vi "Replace Stub SubVIs.vi"(8 "error in":errorcluster, 10 "VIs to Process":path[](array[path]), 11 "subVIs to replace":path[](array[path])) -> (0 "error out":errorcluster)   [LabVIEW 2020, in "NIVS_Consolidated_CDW_MetaDataObj.lvclass"]
uses:
  NIVS_Consolidated_CDW_MetaDataObj.lvclass
  <vilib>/Utility/traverseref.llb/TRef TravTarget.ctl
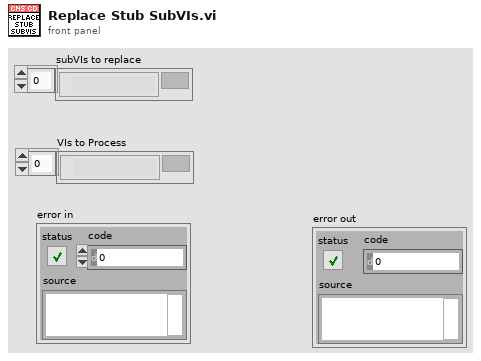
[diagram p1: front panel]
types:
  T1 = typedef "TRef TravTarget.ctl" = enum16{"FP", "BD", "Other"}
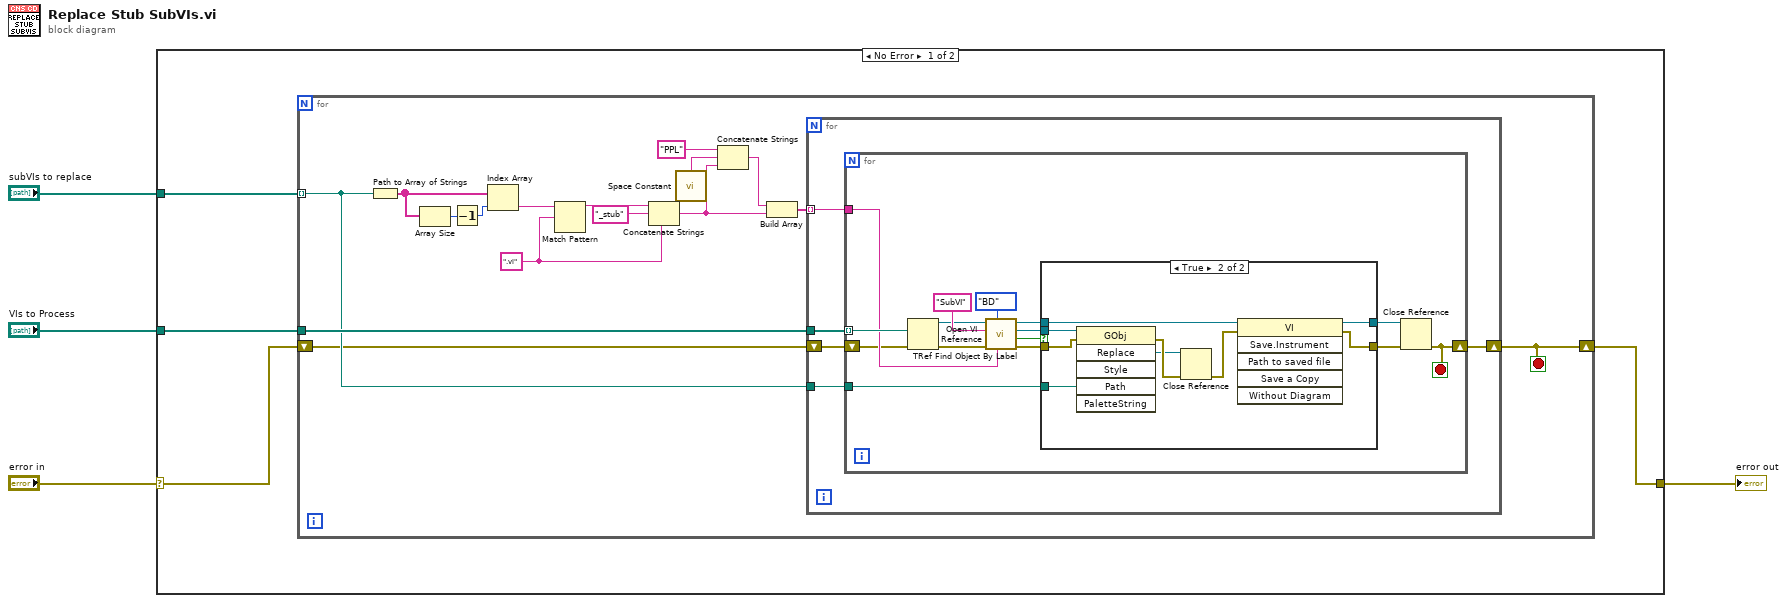
[diagram p0: block diagram]
diagram:
  n1 = case shown="No Error" "error in" {
    selector: "error in" -> [w5 w56]
    tunnel: "VIs to Process" -> [w8 _]
    tunnel: "subVIs to replace" -> [w7 _]
    tunnel: [w6 w56] -> w2
    frame No Error {
      n2 = for {
        tunnel: w7 -> [w16] mode=indexing
        tunnel: w8 -> [w17]
        shift-right: [w14] -> w6
        shift-left: w5 -> [w15]
        stop <- w14 stop-if-true
        w18 = ".vi" ("regular expression")
        n3 = Path to Array of Strings(0:w16) -> (2:w24:string[])  [unwired: 1 out]
        n4 = Array Size(array=w24) -> (size(s)=w23:i32)
        n5 = Decrement(x=w23) -> (x-1=w22:i32)
        n6 = Index Array(array=w24, index=w22) -> (element=w21:string)
        n7 = Match Pattern(string=w21, regular expression=w18) -> (before substring=w20:string)  [unwired: 1 in, 3 out]
        n8 = Concatenate Strings(w20, "_stub" ("string"), w18) -> (w10:string)
        n9 = call <vilib>:"Space Constant.vi"() -> ("String"=w13:string)
        n10 = Concatenate Strings("PPL" ("string"), w13, w10) -> (w11:string)
        n11 = Build Array(w11, w10) -> (w9:string[])
        n12 = for {
          tunnel: w17 -> [w29]
          tunnel: w16 -> [w28]
          shift-right: [w26] -> w14
          shift-left: w15 -> [w27]
          tunnel: w9 -> [w25] mode=indexing
          n13 = for {
            tunnel: w29 -> [w40] mode=indexing
            tunnel: w25 -> [w39]
            tunnel: w28 -> [w36]
            shift-right: [w30] -> w26
            shift-left: w27 -> [w31]
            stop <- w30 stop-if-true
            n14 = Open VI Reference(vi path=w40, error in (no error)=w31) -> (vi reference=w42:refnum<vi>, error out=w41:errorcluster)  [unwired: 4 in]
            n15 = call <vilib>:"TRef Find Object By Label.vi"("Label"=w39, "Traverse Target"=TRef_TravTarget."BD", "error in (no error)"=w41, "Class Name"="SubVI", "VI Ref"=w42) -> ("error out"=w34:errorcluster, "Found?"=w38:bool, "Found Obj Ref"=w37:refnum<vi>, "dup VI Ref"=w35:refnum<vi>)  [unwired: 3 in]
            n16 = case shown="True" w38 {
              tunnel: w37 -> [_ w55]
              tunnel: w36 -> [_ w54]
              tunnel: w35 -> [w46 w53]
              tunnel: w34 -> [w45 w52]
              tunnel: [w46 w49] -> w33
              tunnel: [w45 w48] -> w32
              frame False {
              }
              frame True {
                n17 = invoke class="GObj" method="Replace"(reference=w55, error in=w52, "Path"=w54) -> (error out=w51:errorcluster, "Replace"=w47:refnum<vi>)  [unwired: 3 in, 4 out]
                n18 = Close Reference(reference=w47, error in (no error)=w51) -> (error out=w50:errorcluster)
                n19 = invoke class="VI" method="Save.Instrument"(reference=w53, error in=w50) -> (reference out=w49:refnum<vi>, error out=w48:errorcluster)  [unwired: 4 in, 4 out]
              }
            }
            n20 = Close Reference(reference=w33, error in (no error)=w32) -> (error out=w30:errorcluster)
          }
        }
      }
    }
    frame Error {
    }
  }
  "error out" <- w2
